vi "Explorer Tree Main.vi"(8 "error in (no error)":errorcluster, 10 "Folder Path":path, 11 "TreeControl in":refnum<vi>) -> (0 "error out":errorcluster)   [LabVIEW 2018]
uses:
  <vilib>/Utility/error.llb/DialogType.ctl
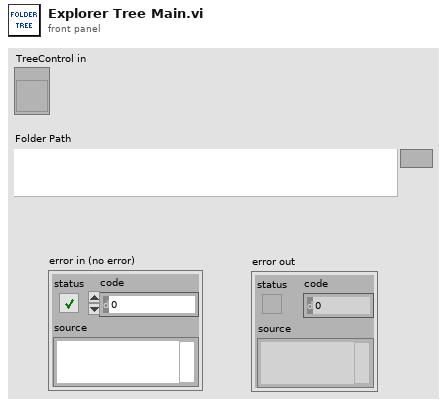
[diagram p1: front panel]
types:
  T1 = typedef "DialogType.ctl" = u16
  T2 = typedef "imagedata.ctl" = cluster{"image type":i32, "image depth":i32, "image":u8[], "mask":u8[], "colors":u32[], "Rectangle":cluster{"left":i16, "top":i16, "right":i16, "bottom":i16}}
  T3 = cluster{"Left Cell String":string, "Child Text":string[], "Child Tag":string, "Item Indent":i32, "Child Only?":bool, "Glyph Index":i32}[]
  T4 = cluster{"Left Cell String":string, "Child Text":string[], "Child Tag":string, "Item Indent":i32, "Child Only?":bool, "Glyph Index":i32}
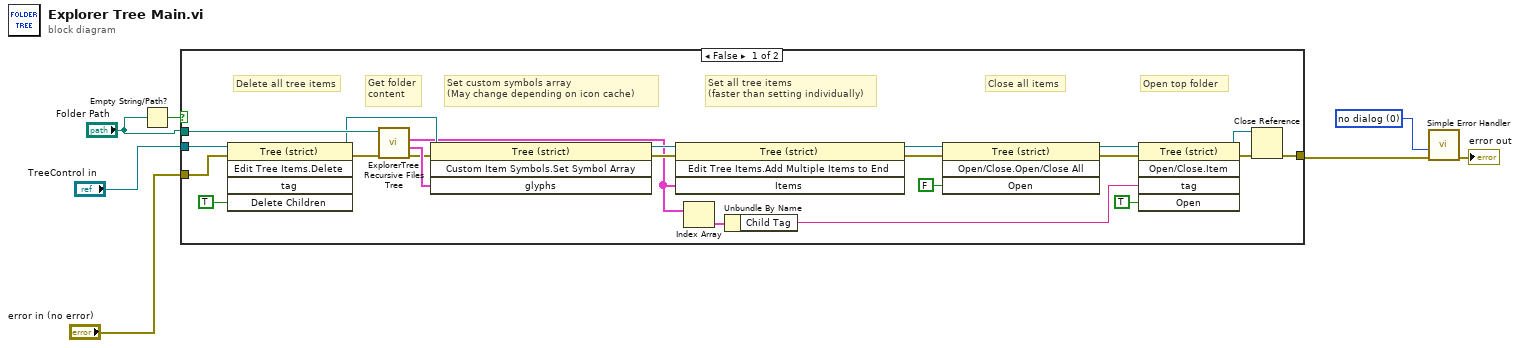
[diagram p0: block diagram]
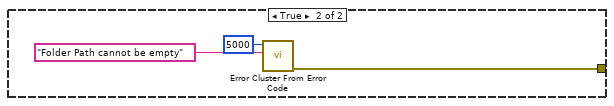
[diagram p2: hidden frame]
diagram:
  w1 = T1 0 items=["no dialog", "OK message", "continue or stop message", "OK message + warnings", "continue/stop + warnings"] ("type of dialog (OK msg:1)")
  n1 = Empty String/Path?(string/path="Folder Path") -> (empty?=w7:bool)
  n2 = case shown="False" w7 {
    tunnel: "TreeControl in" -> [w29 _]
    tunnel: "Folder Path" -> [w26 _]
    tunnel: [w10 w30] -> w5
    tunnel: "error in (no error)" -> [w8 _]
    frame False {
      # "Open top folder"
      # "Close all items"
      # "Set all tree items\n(faster than setting individually)"
      # "Set custom symbols array\n(May change depending on icon cache)"
      # "Get folder\ncontent"
      # "Delete all tree items"
      n3 = invoke class="Tree (strict)" method="Edit Tree Items.Delete"(reference=w29, error in=w8, "Delete Children"=TRUE ("Delete Children?")) -> (reference out=w25:refnum<vi>, error out=w27:errorcluster)  [unwired: 2 in, 3 out]
      n4 = call "ExplorerTree Recursive Files Tree.vi"("error in (no error)"=w27, "Folder Path"=w26) -> ("error out"=w9:errorcluster, "Glyphs"=w24:T2[], "Items"=w16:T3)  [unwired: 6 in, 1 out]
      n5 = invoke class="Tree (strict)" method="Custom Item Symbols.Set Symbol Array"(reference=w25, error in=w9, "glyphs"=w24) -> (reference out=w22:refnum<vi>, error out=w23:errorcluster)  [unwired: 1 in, 2 out]
      n6 = invoke class="Tree (strict)" method="Edit Tree Items.Add Multiple Items to End"(reference=w22, error in=w23, "Items"=w16) -> (reference out=w20:refnum<vi>, error out=w21:errorcluster)  [unwired: 1 in, 2 out]
      n7 = Index Array(array=w16) -> (element=w15:T4)  [unwired: 1 in]
      n8 = Unbundle By Name(w15) -> ("Child Tag"=w14:string)
      n9 = invoke class="Tree (strict)" method="Open/Close.Open/Close All"(reference=w20, error in=w21, "Open"=FALSE ("Open?")) -> (reference out=w18:refnum<vi>, error out=w17:errorcluster)  [unwired: 1 in, 2 out]
      n10 = invoke class="Tree (strict)" method="Open/Close.Item"(reference=w18, error in=w17, "tag"=w14, "Open"=TRUE ("Open?")) -> (reference out=w11:refnum<vi>, error out=w12:errorcluster)  [unwired: 1 in, 3 out]
      n11 = Close Reference(reference=w11, error in (no error)=w12) -> (error out=w10:errorcluster)
    }
    frame True {
      n12 = call <vilib>:"Error Cluster From Error Code.vi"("error message (\"\")"="Folder Path cannot be empty" ("source"), "error code (0)"=5000) -> ("error out"=w30:errorcluster)  [unwired: 7 in]
    }
  }
  n13 = call <vilib>:"Simple Error Handler.vi"("type of dialog (OK msg:1)"=w1, "error in (no error)"=w5) -> ("error out"=→"error out":errorcluster)  [unwired: 3 in, 4 out]
